vi "decision_path.vi"(8 "error in (no error)":errorcluster caption="entrée d'erreur (pas d'erreur)", 11 "ExtraTreesRegressor.lvclass 2":refnum<class "ExtraTreesRegressor.lvclass">) -> (0 "error out":errorcluster caption="sortie d'erreur", 2 "out":T1, 3 "ExtraTreesRegressor.lvclass":refnum<class "ExtraTreesRegressor.lvclass">)   [LabVIEW 2020, in "ExtraTreesRegressor.lvclass"]
doc: "Return the decision path in the forest.\n\n .. versionadded:: 0.18"
uses:
  ExtraTreesRegressor.lvclass
  C:/Users/cipop/TDF Dropbox/2_Technologies de France/1 - Services et Etudes/PLAIY/2 - DEV/PLAIYLAB/code/Python/Python.lvclass
  C:/Users/cipop/TDF Dropbox/2_Technologies de France/1 - Services et Etudes/PLAIY/2 - DEV/PLAIYLAB/code/Model/Model.lvclass
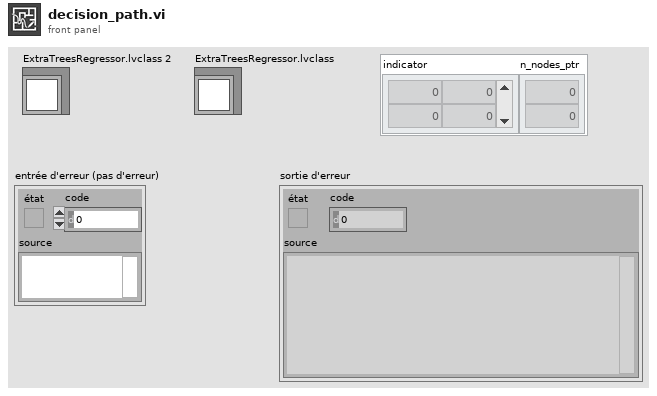
[diagram p1: front panel]
types:
  T1 = cluster{"indicator":dbl[][], "n_nodes_ptr":dbl[]}
  T2 = typedef "data.ctl" = cluster{"name":string, "X":dbl[][]}
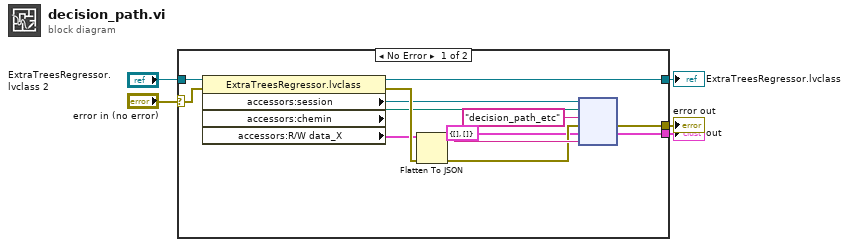
[diagram p0: block diagram]
diagram:
  n1 = case shown="No Error" "error in (no error)" {
    selector: "error in (no error)" -> [w16 w20]
    tunnel: [w17 w20] -> w4
    tunnel: [w9 w19] -> w2
    tunnel: "ExtraTreesRegressor.lvclass 2" -> [w8 w19]
    tunnel: [w6 _] -> w1
    frame No Error {
      n2 = property class="ExtraTreesRegressor.lvclass"(reference=w8, error in=w16) -> (reference out=w9:refnum<class "ExtraTreesRegressor.lvclass">, error out=w14:errorcluster, "accessors:session"=w11:refnum<k35>, "accessors:chemin"=w10:path, "accessors:R/W data_X"=w12:T2)
      n3 = Flatten To JSON(anything=w12, error in (no error)=w14) -> (JSON string=w15:string, 11:w13:errorcluster)  [unwired: 1 in]
      n4 = node(w11, w10, "decision_path_etc" ("nom de la fonction"), w13, T1 {"indicator"=[], "n_nodes_ptr"=[]} ("out"), w15) -> (w17:errorcluster, w6:T1)  [unwired: 1 in, 3 out]
    }
    frame Error {
    }
  }
  "error out" <- w4
  "ExtraTreesRegressor.lvclass" <- w2
  "out" <- w1
